vi "Disconnect.vi"(8 "error in (no error)":errorcluster, 11 "Picomotor8742Comm in":refnum<class "TCPCommClass.lvclass">) -> (0 "error out":errorcluster, 3 "Picomotor8742Comm out":refnum<class "TCPCommClass.lvclass">)   [LabVIEW 2013, in "TCPCommClass.lvclass"]
uses:
  TCPCommClass.lvclass
  TCPCommClass.lvclass/TCPCommClass.ctl
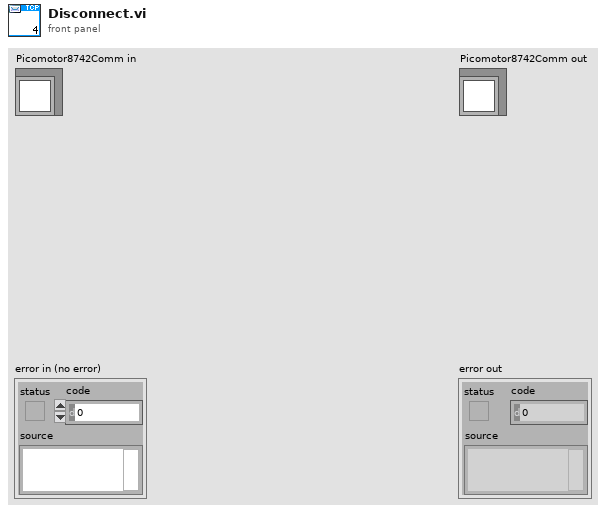
[diagram p1: front panel]
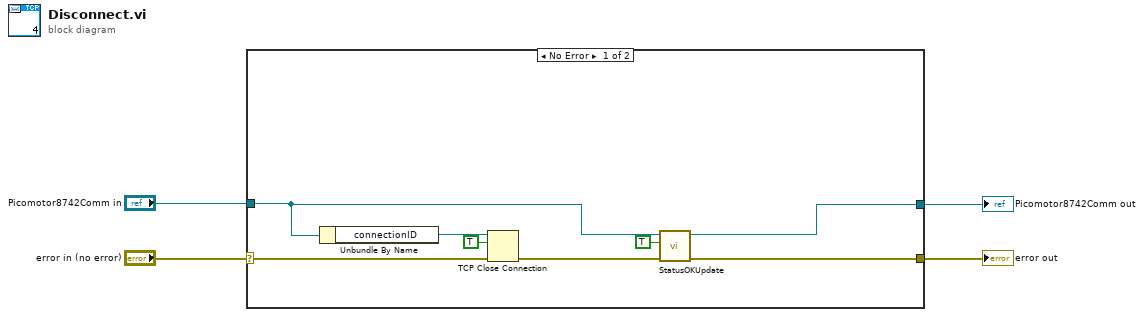
[diagram p0: block diagram]
diagram:
  n1 = case shown="No Error" "error in (no error)" {
    selector: "error in (no error)" -> [w12 w14]
    tunnel: [w7 w14] -> w3
    tunnel: [w5 w13] -> w1
    tunnel: "Picomotor8742Comm in" -> [w9 w13]
    frame No Error {
      n2 = Unbundle By Name(w9) -> ("connectionID"=w11:refnum<k5>)
      n3 = TCP Close Connection(connection ID=w11, abort (F)=TRUE, error in (no error)=w12) -> (error out=w8:errorcluster)  [unwired: 1 out]
      n4 = call-dynamic "StatusOKUpdate.vi"("error in (no error)"=w8, "OkIn"=TRUE, "Picomotor8742Comm in"=w9) -> ("error out"=w7:errorcluster, "Picomotor8742Comm out"=w5:refnum<class "TCPCommClass.lvclass">)  [unwired: 7 in]
    }
    frame Error {
    }
  }
  "error out" <- w3
  "Picomotor8742Comm out" <- w1
